vi "Msg.Noti.Wait.vi"(8 "Error (in)":errorcluster, 11 "Msg.Refs":T1) -> (0 "Error (out)":errorcluster, 1 "Data":variant, 2 "Message":string, 3 "Msg.Refs (out)":T1)   [LabVIEW 2023, in "MessagingModule.lvlib"]
uses:
  MessagingModule.lvlib
  Msg.Data.ctl
  Msg.Event.Ref.ctl
  Msg.Event.RegRef.ctl
  Msg.Q.Ref.ctl
  Msg.Noti.Ref.ctl
  Msg.Refs.ctl
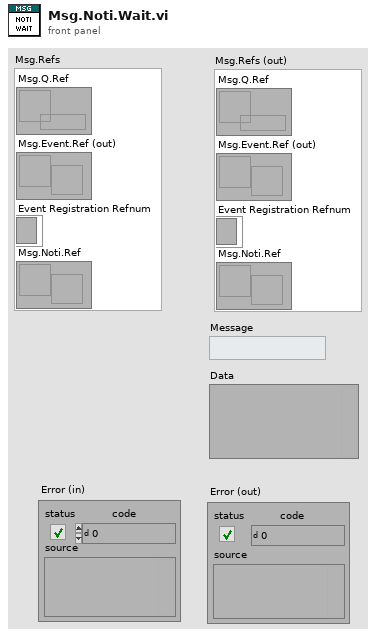
[diagram p1: front panel]
types:
  T1 = typedef "MessagingModule.lvlib/Msg.Refs.ctl" = cluster{"Msg.Q.Ref":T2, "Msg.Event.Ref (out)":T3, "Event Registration Refnum":T4, "Msg.Noti.Ref":T5}
  T2 = typedef "MessagingModule.lvlib/Msg.Q.Ref.ctl" = refnum<queue>
  T3 = typedef "MessagingModule.lvlib/Msg.Event.Ref.ctl" = refnum<user-event>
  T4 = typedef "MessagingModule.lvlib/Msg.Event.RegRef.ctl" = refnum<event-registration>
  T5 = typedef "MessagingModule.lvlib/Msg.Noti.Ref.ctl" = refnum<notifier>
  T6 = typedef "MessagingModule.lvlib/Msg.Data.ctl" = cluster{"Message":string, "Data":variant}
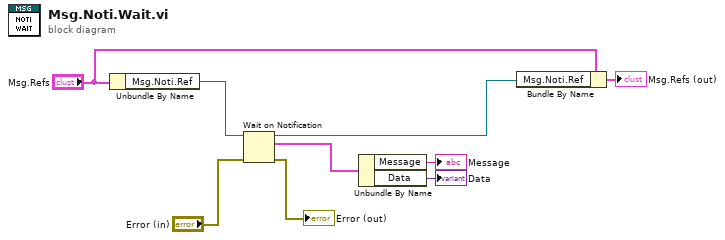
[diagram p0: block diagram]
diagram:
  n1 = Unbundle By Name("Msg.Refs") -> ("Msg.Noti.Ref"=w4:T5)
  n2 = Wait on Notification(notifier=w4, error in (no error)="Error (in)") -> (notifier out=w3:T5, notification=w7:T6, error out=→"Error (out)":errorcluster)  [unwired: 2 in, 1 out]
  n3 = Unbundle By Name(w7) -> ("Message"=→"Message":string, "Data"=→"Data":variant)
  n4 = Bundle By Name(cluster="Msg.Refs", "Msg.Noti.Ref"=w3) -> (→"Msg.Refs (out)":T1)
